vi "Update folder size.vi"(8 "error in (no error)":errorcluster, 11 "Folder in":refnum<class "Folder.lvclass">) -> (0 "error out":errorcluster, 2 "Contained size":i32, 3 "Folder out":refnum<class "Folder.lvclass">)   [LabVIEW 2020, in "Folder.lvclass"]
uses:
  Folder.lvclass
  Folder.lvclass/Folder.ctl
  system object/system object.lvclass
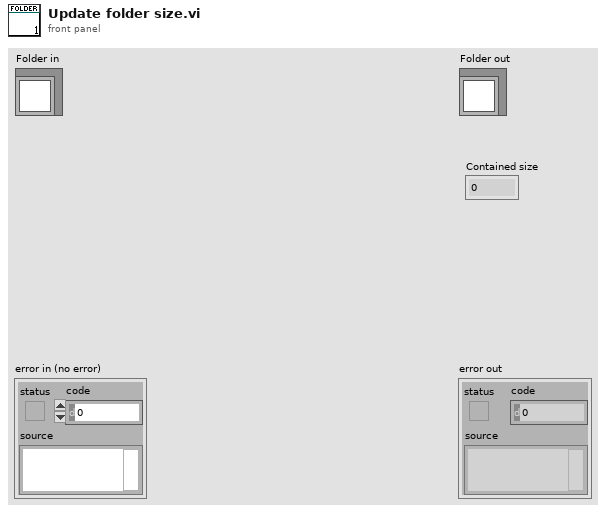
[diagram p1: front panel]
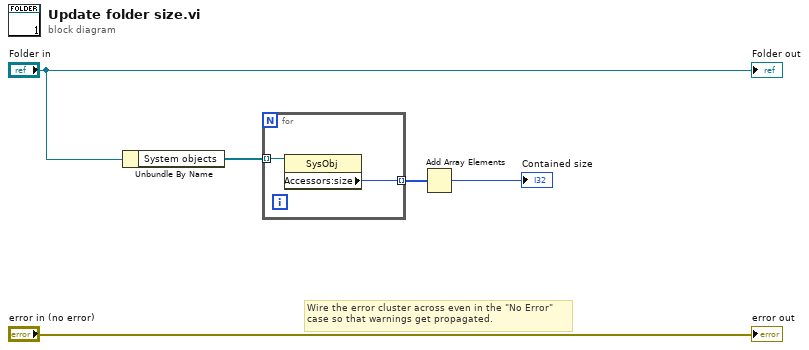
[diagram p0: block diagram]
diagram:
  # "Wire the error cluster across even in the \"No Error\"\ncase so that warnings get propagated."
  n1 = Unbundle By Name("Folder in") -> ("System objects"=w3:refnum<class "system object.lvclass">[])
  n2 = for {
    tunnel: w3 -> [w7] mode=indexing
    tunnel: [w6] -> w2 mode=indexing
    n3 = property class="SysObj"(reference=w7) -> ("Accessors:size"=w6:i32)  [unwired: 1 in, 2 out]
  }
  n4 = Add Array Elements(numeric array=w2) -> (sum=→"Contained size":i32)
  "error out" <- "error in (no error)"
  "Folder out" <- "Folder in"
